vi "main.vi"() -> ()   [LabVIEW 2015]
uses:
  Controls/TDE_Type_2.ctl
  <vilib>/Utility/error.llb/DialogType.ctl
  <vilib>/Utility/file.llb/Write Delimited Spreadsheet (string).vi
panel:
  in  "export":bool
  out "stats":cluster{i32, T1}[](array[cluster])
  out "sum-up":cluster{timestamp, T1}[](array[cluster]) {"?" format="%<%Y.%m.%d %Hh%Mm%S%3u>T"}
  in  "Path":path
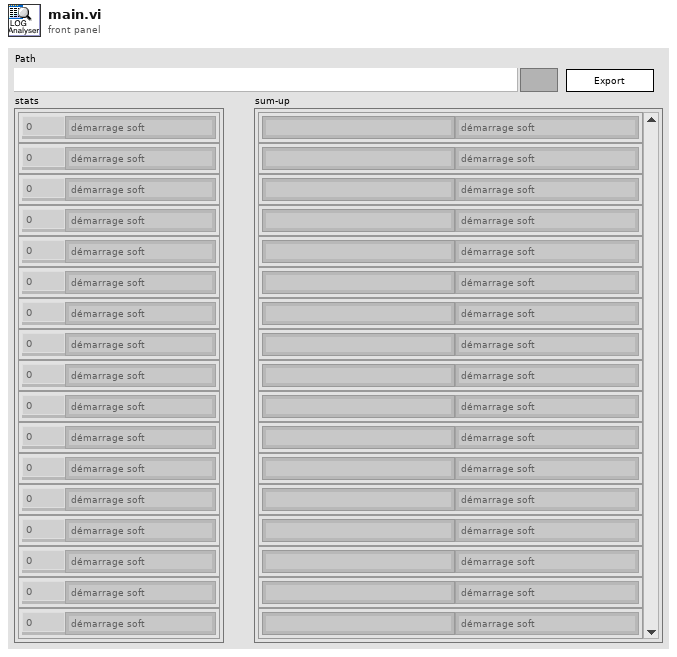
[diagram p1: front panel]
types:
  T1 = typedef "TDE_Type_2.ctl" = enum8{"démarrage soft", "start prod", "Mire", "start cames", "stop cames", "RàZ Vision", "en marche", "P2 ok", "acqFail embout", "acqFail profil", "acqFail collerette", "error open", "error get image", "error 2", "error 3", "error 4", "error 5", "autre"}
  T2 = cluster{"config file":path, "default folder":path, "current file":path, "lines":string[], "full story":cluster{timestamp, T1}[], "sum-up":cluster{timestamp, T1}[], "stats":cluster{i32, T1}[]}
  T3 = enum16{"open", "replace", "create", "open or create", "replace or create", "replace or create with confirmation"}
  T4 = typedef "DialogType.ctl" = u16
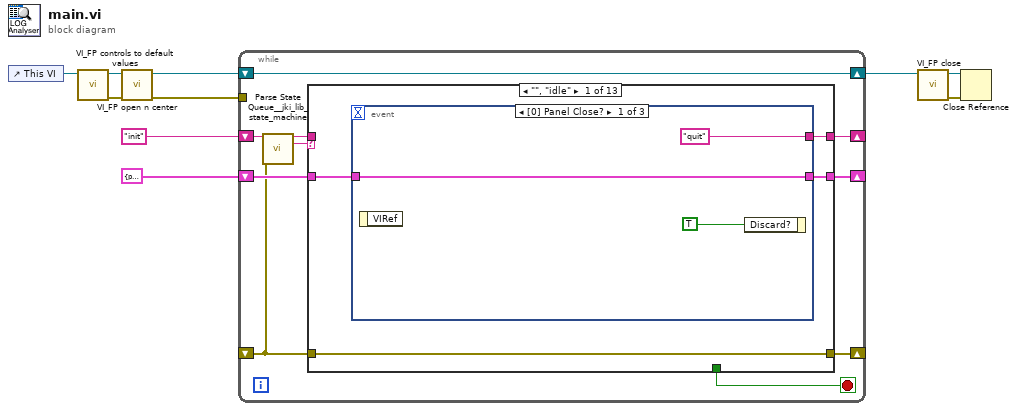
[diagram p0: block diagram]
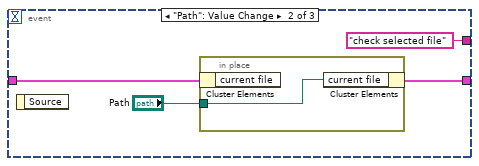
[diagram p2: hidden frame]
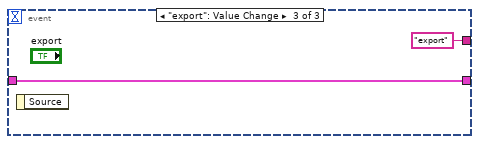
[diagram p3: hidden frame]
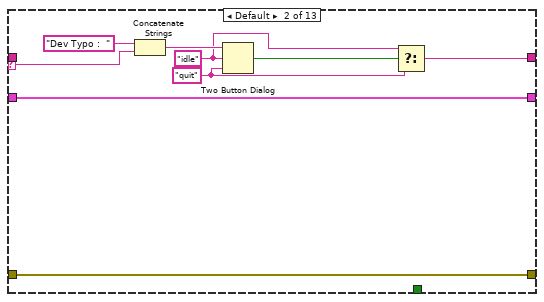
[diagram p4: hidden frame]
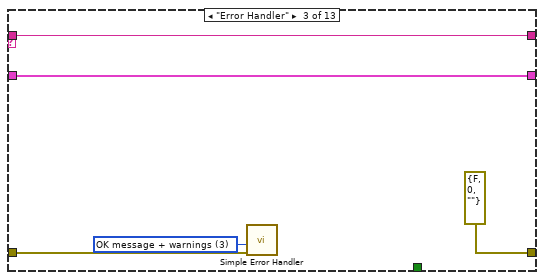
[diagram p5: hidden frame]
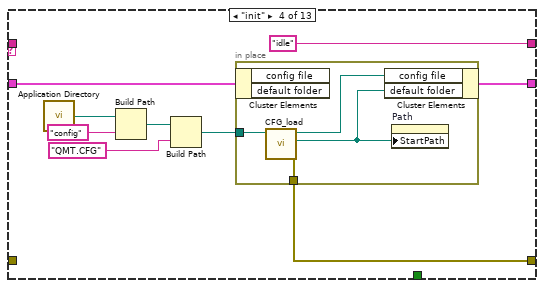
[diagram p6: hidden frame]
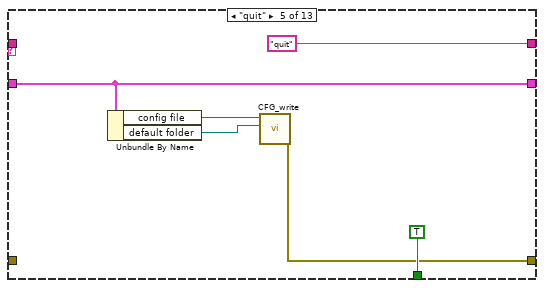
[diagram p7: hidden frame]
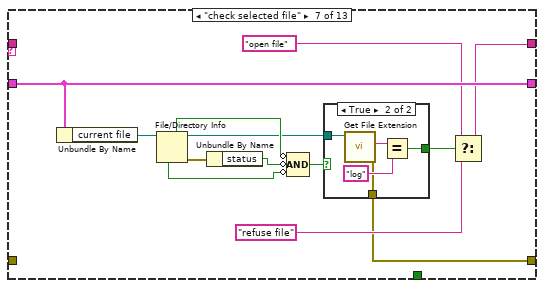
[diagram p9: hidden frame]
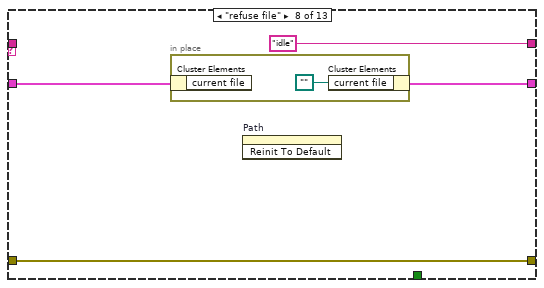
[diagram p11: hidden frame]
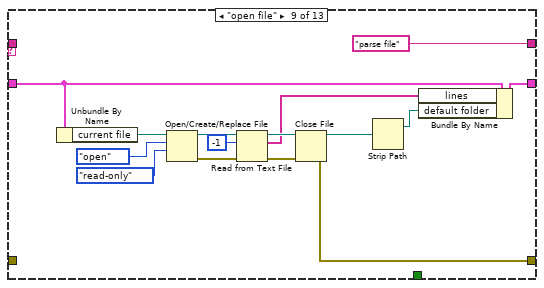
[diagram p12: hidden frame]
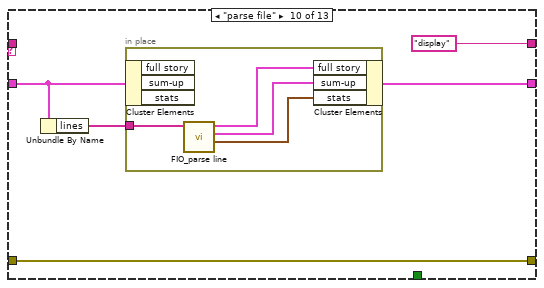
[diagram p13: hidden frame]
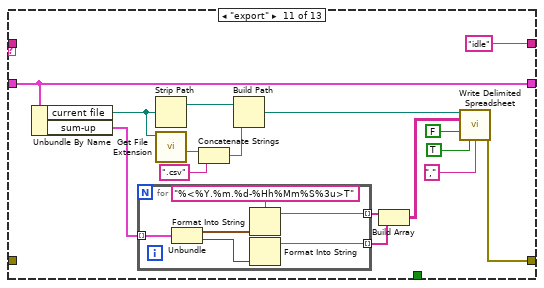
[diagram p14: hidden frame]
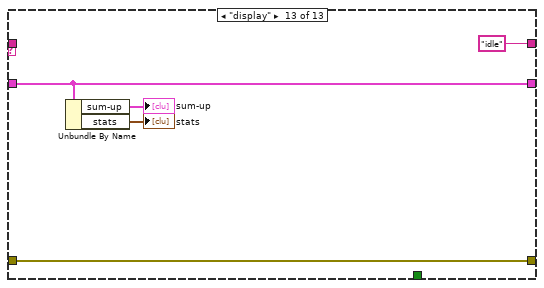
[diagram p16: hidden frame]
diagram:
  n1 = control-ref of="This VI"() -> (w10:refnum<vi>)
  n2 = call "VI_FP controls to default values.vi"("VI in"=w10) -> ("error out"=w7:errorcluster, "VI out"=w9:refnum<vi>)  [unwired: 9 in]
  n3 = call "VI_FP open n center.vi"("error in (no error)"=w7, "VI in"=w9) -> ("error out"=w6:errorcluster, "VI out"=w8:refnum<vi>)  [unwired: 8 in]
  n4 = while {
    shift-right: [w19] -> w5
    shift-left: w8 -> [w19]
    tunnel: w6 -> [_]
    shift-right: [w17] -> _
    shift-left: T2 {"config file"=path "", "default folder"=path "", "current file"=path "", "lines"=[], "full story"=[], "sum-up"=[], "stats"=[]} -> [w18]
    shift-right: [w16] -> _
    shift-left: "init" -> [w15]
    shift-right: [w13] -> _
    shift-left: _ -> [w11]
    stop <- w20 stop-if-true
    n5 = call <vilib>:"Parse State Queue__jki_lib_state_machine.vi"("State Queue"=w15, "Error In (no error)"=w11) -> ("Remaining States"=w12:string, "Current State"=w14:string)  [unwired: 11 in, 1 out]
    n6 = case shown="\"\", \"idle\"" w14 {
      selector: w14 -> [_ w42 _ _ _ w70 _ _ _ _ _ w142 _]
      tunnel: [_ _ _ _ TRUE ("Discard?") _ _ _ _ _ _ _ _] -> w20
      tunnel: w18 -> [w24 w43 w48 w52 w65 w69 w83 w91 w100 w111 w132 w141 w146]
      tunnel: [w23 w43 w48 w51 w65 w69 w83 w90 w99 w110 w132 w141 w146] -> w17
      tunnel: [w22 w36 w47 "idle" "quit" w70 w75 "idle" "parse file" ("f") "display" "idle" w142 "idle"] -> w16
      tunnel: [w21 w35 errorcluster {"status"=FALSE, "code"=0, "source"=""} ("error out") w49 w62 w68 w71 w89 w94 w109 w118 w140 w143] -> w13
      tunnel: w12 -> [_ _ w47 _ _ _ _ _ _ _ _ _ _]
      tunnel: w11 -> [w21 w35 w46 _ _ w68 _ w89 _ w109 _ w140 w143]
      frame "", "idle" {
        n7 = event shown="[0] Panel Close?" {
          selector: _ -> [_ _ _]
          dyn-events: _ -> [_ _ _]
          timeout: _ -> [_ _ _]
          tunnel: w24 -> [w26 w31 w34]
          tunnel: [w26 w30 w34] -> w23
          tunnel: ["quit" "check selected file" "export"] -> w22
          event Panel Close? {
            n8 = event-data() -> ()  [unwired: 1 in, 1 out]
            n9 = event-data("Discard?"=TRUE) -> ()  [unwired: 1 in, 1 out]
          }
          event "Path": Value Change {
            n10 = event-data() -> ()  [unwired: 1 in, 1 out]
            n11 = in-place {
              in-place-border: "Path" -> [w32]
              n12 = in-place-cluster #1(w31) -> ()  [unwired: 1 out]
              n13 = in-place-cluster #1("current file"=w32) -> (w30:T2)
            }
          }
          event "export": Value Change {
            n14 = event-data() -> ()  [unwired: 1 in, 1 out]
          }
        }
      }
      frame Default {
        w37 = "quit"
        w38 = "idle"
        n15 = Concatenate Strings("Dev Typo :  " ("button name (\"OK\")"), w42) -> (w40:string)
        n16 = Two Button Dialog(message=w40, 1:w37, 2:w38) -> (T button?=w39:bool)
        n17 = Select(t=w38, s=w39, f=w37) -> (s? t:f=w36:string)
      }
      frame "Error Handler" {
        w45 = T4 3 items=["no dialog", "OK message", "continue or stop message", "OK message + warnings", "continue/stop + warnings"] ("type of dialog (OK msg:1)")
        n18 = call <vilib>:"Simple Error Handler.vi"("type of dialog (OK msg:1)"=w45, "error in (no error)"=w46) -> ()  [unwired: 3 in, 5 out]
      }
      frame "init" {
        n19 = call <vilib>:"Application Directory.vi"() -> ("Application Directory"=w56:path)
        n20 = Build Path(base path=w56, name or relative path="config") -> (appended path=w54:path)
        n21 = Build Path(base path=w54, name or relative path="QMT.CFG") -> (appended path=w50:path)
        n22 = in-place {
          in-place-border: w50 -> [w61]
          in-place-border: [w58] -> w49
          n23 = in-place-cluster #2(w52) -> ()  [unwired: 2 out]
          n24 = call "CFG_load.vi"("config file"=w61) -> ("error out"=w58:errorcluster, "default folder"=w59:path, "config file dup"=w60:path)  [unwired: 8 in]
          n25 = in-place-cluster #2("config file"=w60, "default folder"=w59) -> (w51:T2)
          n26 = property on="Path" class="Path"("StartPath"=w59) -> ()  [unwired: 2 in, 2 out]
        }
      }
      frame "quit" {
        n27 = Unbundle By Name(w65) -> ("config file"=w64:path, "default folder"=w63:path)
        n28 = call "CFG_write.vi"("default folder"=w63, "config file"=w64) -> ("error out"=w62:errorcluster)  [unwired: 8 in, 1 out]
      }
      frame "----------File---------- " {
      }
      frame "check selected file" {
        n29 = Unbundle By Name(w83) -> ("current file"=w82:path)
        n30 = File/Directory Info(path=w82) -> (path out=w73:path, directory=w81:bool, error out=w79:errorcluster, shortcut=w80:bool)  [unwired: 1 in, 3 out]
        n31 = Unbundle By Name(w79) -> ("status"=w78:bool)
        n32 = Compound Arithmetic op=AND(invert w81, invert w78, invert w80) -> (w74:bool)
        n33 = case shown="True" w74 {
          tunnel: w73 -> [_ w88]
          tunnel: [_ w85] -> w72
          tunnel: [_ w84] -> w71
          frame False {
          }
          frame True {
            n34 = call <vilib>:"Get File Extension.vi"("file"=w88) -> ("error out"=w84:errorcluster, "lowercase file extension"=w87:string)  [unwired: 6 in, 3 out]
            n35 = Equal?(x=w87, y="log") -> (x = y?=w85:bool)
          }
        }
        n36 = Select(t="open file", s=w72, f="refuse file") -> (s? t:f=w75:string)
      }
      frame "refuse file" {
        n37 = in-place {
          n38 = in-place-cluster #3(w91) -> ()  [unwired: 1 out]
          n39 = in-place-cluster #3("current file"=path "") -> (w90:T2)
        }
        n40 = invoke on="Path" class="Path" method="Reinit To Default"() -> ()  [unwired: 3 in, 3 out]
      }
      frame "open file" {
        n41 = Unbundle By Name(w100) -> ("current file"=w108:path)
        n42 = Open/Create/Replace File(file path (use dialog)=w108, operation (0:open)=T3."open", access (0:read/write)=enum16{"read/write", "read-only", "write-only"}."read-only") -> (refnum out=w106:refnum<file>, error out=w107:errorcluster)  [unwired: 3 in, 1 out]
        n43 = Read from Text File(file (use dialog)=w106, count=-1, error in=w107) -> (refnum out=w101:refnum<file>, text=w98:string[], error out=w102:errorcluster)  [unwired: 1 in, 1 out]
        n44 = Close File(refnum=w101, error in=w102) -> (path=w97:path, error out=w94:errorcluster)
        n45 = Strip Path(path=w97) -> (stripped path=w96:path)  [unwired: 1 out]
        n46 = Bundle By Name(cluster=w100, "lines"=w98, "default folder"=w96) -> (w99:T2)
      }
      frame "parse file" {
        n47 = Unbundle By Name(w111) -> ("lines"=w112:string[])
        n48 = in-place {
          in-place-border: w112 -> [w117]
          n49 = in-place-cluster #4(w111) -> ()  [unwired: 3 out]
          n50 = call "FIO_parse line.vi"("lines"=w117) -> ("stats"=w114:cluster{i32, T1}[], "sum-up"=w115:cluster{timestamp, T1}[], "full story"=w116:cluster{timestamp, T1}[])  [unwired: 8 in]
          n51 = in-place-cluster #4("full story"=w116, "sum-up"=w115, "stats"=w114) -> (w110:T2)
        }
      }
      frame "export" {
        n52 = Unbundle By Name(w132) -> ("current file"=w130:path, "sum-up"=w123:cluster{timestamp, T1}[])
        n53 = for {
          tunnel: w123 -> [w139] mode=indexing
          tunnel: [w136] -> w122 mode=indexing
          tunnel: [w134] -> w121 mode=indexing
          n54 = Unbundle(w139) -> (w138:timestamp, w135:T1)
          n55 = Format Into String(format string="%<%Y.%m.%d-%Hh%Mm%S%3u>T", w138) -> (resulting string=w136:string)  [unwired: 2 in, 1 out]
          n56 = Format Into String(w135) -> (resulting string=w134:string)  [unwired: 3 in, 1 out]
        }
        n57 = Strip Path(path=w130) -> (stripped path=w131:path)  [unwired: 1 out]
        n58 = call <vilib>:"Get File Extension.vi"("file"=w130) -> ("filename without extension"=w129:string)  [unwired: 6 in, 4 out]
        n59 = Concatenate Strings(w129, ".csv" ("string")) -> (w127:string)
        n60 = Build Path(base path=w131, name or relative path=w127) -> (appended path=w126:path)
        n61 = Build Array(w122, w121) -> (w120:string[][])
        n62 = call-poly <vilib>:"Write Delimited Spreadsheet.vi"("file path (dialog if empty)"=w126, "2D data"=w120, "append to file? (F)"=FALSE, "transpose? (F)"=TRUE, "delimiter (\\t)"="," ("delimiter (\\t)")) -> ("error out"=w118:errorcluster)  [unwired: 9 in, 1 out]
      }
      frame "----------UI---------- " {
      }
      frame "display" {
        n63 = Unbundle By Name(w146) -> ("sum-up"=→"sum-up":cluster{timestamp, T1}[], "stats"=→"stats":cluster{i32, T1}[])
      }
    }
  }
  n64 = call "VI_FP close.vi"("VI in"=w5) -> ("error out"=w4:errorcluster, "VI out"=w3:refnum<vi>)  [unwired: 9 in]
  n65 = Close Reference(reference=w3, error in (no error)=w4) -> ()  [unwired: 1 out]
